vi "аналогові.vi"() -> ()   [LabVIEW 2013]
uses:
  <vilib>/DAQmx/write.llb/DAQmx Write (Analog DBL 1Chan 1Samp).vi
  <vilib>/DAQmx/read.llb/DAQmx Read (Analog DBL 1Chan 1Samp).vi
  <vilib>/DAQmx/create/channels.llb/DAQmx Create Channel (AI-Voltage-Basic).vi
  <vilib>/DAQmx/create/channels.llb/DAQmx Create Channel (AO-Voltage-Basic).vi
  <vilib>/DAQmx/miscellaneous.llb/DAQmx Fill In Error Info.vi
panel:
  in  "stop":bool
  in  "запис":dbl min=0.0 max=5.0 step=1.0 format="%0.2f"
  out "зчитування":dbl format="%0.2f"
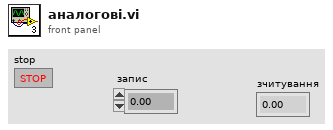
[diagram p1: front panel]
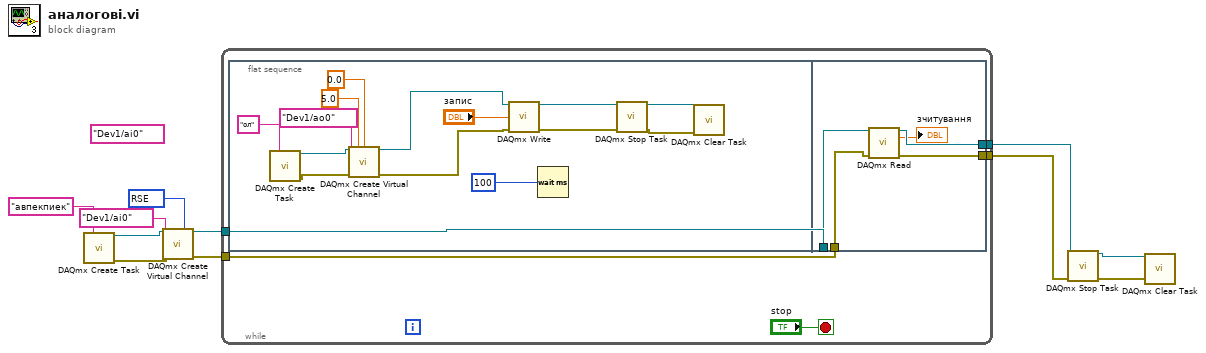
[diagram p0: block diagram]
diagram:
  w1 = 10083 items=["default"=-1, "RSE"=10083, "NRSE"=10078, "Differential"=10106, "Pseudodifferential"=12529] ("input terminal configuration")
  (unwired) tag "Dev1/ai0" ("physical channels")
  n1 = call <vilib>:"DAQmx Create Task.vi"("new task name"="авпекпиек") -> ("task out"=w11:refnum<k21>, "error out"=w8:errorcluster)  [unwired: 13 in]
  n2 = call-poly <vilib>:"DAQmx Create Virtual Channel.vi"("task in"=w11, "input terminal configuration"=w1, "physical channels"=tag "Dev1/ai0", "error in"=w8) -> ("task out"=w10:refnum<k21>, "error out"=w7:errorcluster)  [unwired: 10 in]
  n3 = while {
    tunnel: w10 -> [w16]
    tunnel: w7 -> [w15]
    tunnel: [w14] -> w6
    tunnel: [w13] -> w3
    stop <- "stop" stop-if-true
    n4 = flat-sequence {
      tunnel: w16 -> [w35]
      tunnel: w15 -> [w34]
      tunnel: [w33] -> w14
      tunnel: [w32] -> w13
      frame #0 {
        n5 = call <vilib>:"DAQmx Create Task.vi"("new task name"="ол") -> ("task out"=w23:refnum<k21>, "error out"=w26:errorcluster)  [unwired: 13 in]
        n6 = call-poly <vilib>:"DAQmx Create Virtual Channel.vi"("task in"=w23, "maximum value"=5.0, "minimum value"=0.0, "physical channels"=tag "Dev1/ao0", "error in"=w26) -> ("task out"=w22:refnum<k21>, "error out"=w21:errorcluster)  [unwired: 9 in]
        n7 = call-poly <vilib>:"DAQmx Write.vi"("task/channels in"=w22, "data"="запис", "error in"=w21) -> ("task out"=w18:refnum<k21>, "error out"=w17:errorcluster)  [unwired: 10 in, 1 out]
        n8 = Wait (ms)(milliseconds to wait=u32 100) -> ()  [unwired: 1 out]
        n9 = call <vilib>:"DAQmx Stop Task.vi"("task/channels in"=w18, "error in"=w17) -> ("task out"=w19:refnum<k21>, "error out"=w20:errorcluster)  [unwired: 12 in]
        n10 = call <vilib>:"DAQmx Clear Task.vi"("task in"=w19, "error in"=w20) -> ()  [unwired: 13 in, 1 out]
      }
      frame #1 {
        n11 = call-poly <vilib>:"DAQmx Read.vi"("task/channels in"=w35, "error in"=w34) -> ("task out"=w32:refnum<k21>, "data"=→"зчитування":dbl, "error out"=w33:errorcluster)  [unwired: 11 in]
      }
    }
  }
  n12 = call <vilib>:"DAQmx Stop Task.vi"("task/channels in"=w3, "error in"=w6) -> ("task out"=w4:refnum<k21>, "error out"=w5:errorcluster)  [unwired: 12 in]
  n13 = call <vilib>:"DAQmx Clear Task.vi"("task in"=w4, "error in"=w5) -> ()  [unwired: 13 in, 1 out]
